vi "roboRIO v1.0 Open Relay.vi"(7 "Allow multiple opens?":bool, 8 "error in (no error)":errorcluster, 10 "Channel Names":string[](array[string]), 11 "Resource name":T3 caption="RIO Device") -> (0 "error out":errorcluster, 2 "Relay Channel List":T4, 3 "myRIO Ref Out":T1)   [LabVIEW 2021]
uses:
  <vilib>/myRIO/Common/Instrument Driver Framework/roboRIO v1.0/Relay/typedefs/Relay Channels List.ctl
  <vilib>/myRIO/Common/Instrument Driver Framework/roboRIO v1.0/Relay/typedefs/Relay Channels Enum.ctl
  <vilib>/userDefined/High Color/nirio_resource_hc.ctl
  <vilib>/myRIO/Common/Instrument Driver Framework/Utilities/typedefs/myRIO v1.0 Reference.ctl
  <vilib>/myRIO/Common/Instrument Driver Framework/Utilities/typedefs/Generic FPGA Reference.ctl
  <vilib>/myRIO/Common/Instrument Driver Framework/roboRIO v1.0/Resource Manager/vis/roboRIO v1.0 Reserve Channel List.vi
  <vilib>/myRIO/Common/Instrument Driver Framework/roboRIO v1.0/Relay/vis/roboRIO v1.0 Build MUX Configuration Relay.vi
  <vilib>/myRIO/Common/Instrument Driver Framework/roboRIO v1.0/Resource Manager/vis/roboRIO v1.0 Reserve Channel.vi
  <vilib>/myRIO/Common/Instrument Driver Framework/roboRIO v1.0/Resource Manager/vis/roboRIO v1.0 Unreserve Channel.vi
  <vilib>/myRIO/Common/Instrument Driver Framework/roboRIO v1.0/Resource Manager/vis/roboRIO v1.0 Build Mutex Name.vi
  <vilib>/Utility/VariantDataType/GetNumericInfo.vi
  <vilib>/Utility/error.llb/Error Cluster From Error Code.vi
  <vilib>/myRIO/Common/Instrument Driver Framework/Utilities/vis/IO Manager.vi
  <vilib>/myRIO/Common/Instrument Driver Framework/Utilities/vis/Configuration Manager.vi
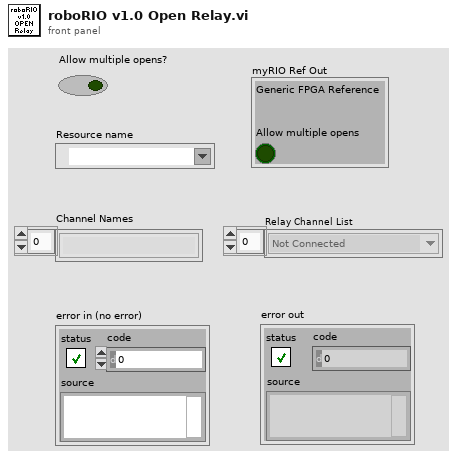
[diagram p1: front panel]
types:
  T1 = typedef "myRIO v1.0 Reference.ctl" = cluster{"Generic FPGA Reference":T2, "Allow multiple opens":bool}
  T2 = typedef "Generic FPGA Reference.ctl" = refnum<k20>
  T3 = typedef "nirio_resource_hc.ctl" = tag
  T4 = typedef "Relay Channels List.ctl" = T5[]
  T5 = typedef "Relay Channels Enum.ctl" = enum16{"Not Connected", "RELAY/RELAY0", "RELAY/RELAY1", "RELAY/RELAY2", "RELAY/RELAY3"}
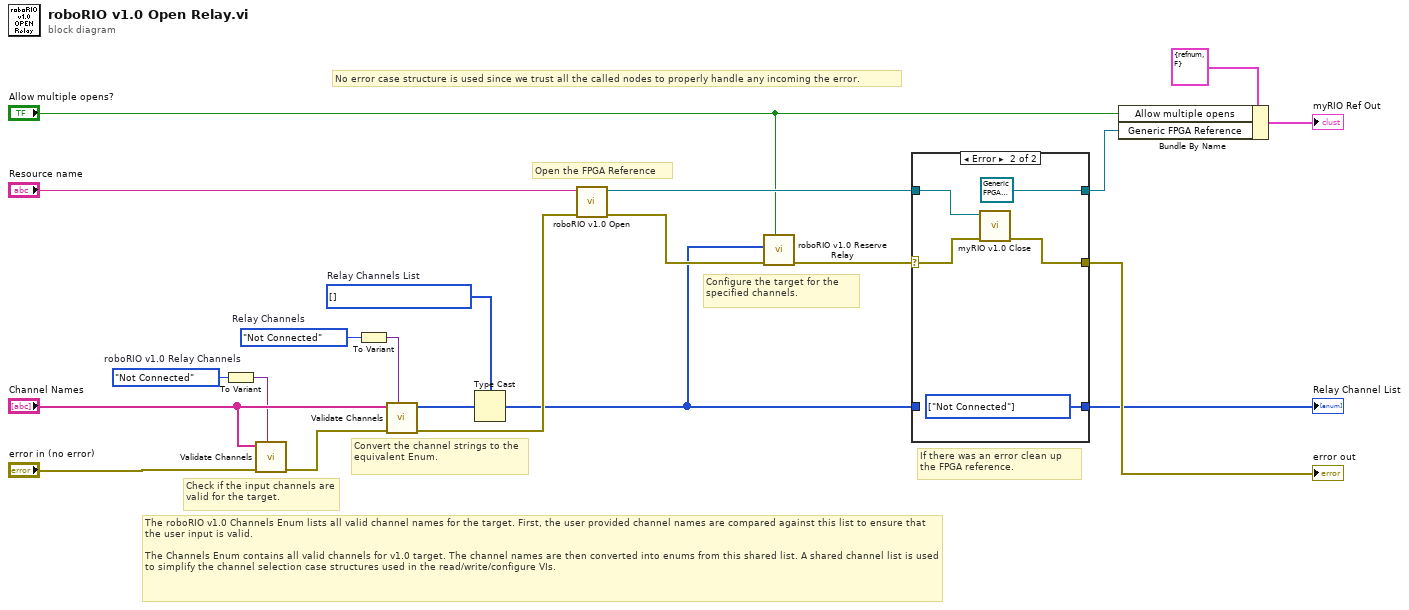
[diagram p0: block diagram]
diagram:
  w2 = Relay_Channels_Enum."Not Connected"  # Relay Channels
  w1 = Relay_Channels_Enum."Not Connected"  # roboRIO v1.0 Relay Channels
  w15 = T4 [] items=["Not Connected", "RELAY/RELAY0", "RELAY/RELAY1", "RELAY/RELAY2", "RELAY/RELAY3"]  # Relay Channels List
  # "The roboRIO v1.0 Channels Enum lists all valid channel names for the target. First, the user provided channel names are compared against this list to ensure that the user input is valid.\n\nThe Channels Enum contains all valid channels for v1.0 target. The channel names are then converted into enums from this shared list. A shared channel list is used to simplify the channel selection case structures used in the read/write/configure VIs."
  # "If there was an error clean up the FPGA reference."
  # "Configure the target for the specified channels."
  # "Open the FPGA Reference"
  # "No error case structure is used since we trust all the called nodes to properly handle any incoming the error."
  # "Convert the channel strings to the equivalent Enum."
  # "Check if the input channels are valid for the target."
  n1 = To Variant(anything=w1) -> (Variant=w3:variant)
  n2 = call <vilib>:"Validate Channels.vi"("Channels Enum Variant"=w3, "error in (no error)"="error in (no error)", "Channel Names"="Channel Names") -> ("error out"=w20:errorcluster)  [unwired: 7 in, 1 out]
  n3 = To Variant(anything=w2) -> (Variant=w4:variant)
  n4 = call <vilib>:"Validate Channels.vi"("Channels Enum Variant"=w4, "error in (no error)"=w20, "Channel Names"="Channel Names") -> ("error out"=w16:errorcluster, "Index Array"=w14:u16[])  [unwired: 7 in]
  n5 = Type Cast(type=w15, x=w14) -> (*(type *) &x=w10:T4)
  n6 = call <vilib>:"roboRIO v1.0 Open.vi"("error in (no error)"=w16, "Resource name"="Resource name") -> ("error out"=w13:errorcluster, "myRIO FPGA Ref Out"=w11:T2)  [unwired: 8 in]
  n7 = call <vilib>:"roboRIO v1.0 Reserve Relay.vi"("Allow multiple opens?"="Allow multiple opens?", "error in (no error)"=w13, "Relay Channel List"=w10) -> ("error out"=w12:errorcluster)  [unwired: 8 in]
  n8 = case shown="Error" w12 {
    selector: w12 -> [w23 w29]
    tunnel: w11 -> [w24 w27]
    tunnel: [w24 T2 refnum ("roboRIO FPGA Ref Out")] -> w6
    tunnel: [w23 w28] -> w18
    tunnel: w10 -> [w22 _]
    tunnel: [w22 w25] -> w9
    frame No Error {
    }
    frame Error {
      w25 = T4 [enum."Not Connected"] items=["Not Connected", "RELAY/RELAY0", "RELAY/RELAY1", "RELAY/RELAY2", "RELAY/RELAY3"] ("DIO Channels List")
      n9 = call <vilib>:"myRIO v1.0 Close.vi"("error in (no error)"=w29, "myRIO FPGA Ref In"=w27) -> ("error out"=w28:errorcluster)  [unwired: 9 in]
    }
  }
  "Relay Channel List" <- w9
  "error out" <- w18
  n10 = Bundle By Name(cluster=T1 {"Generic FPGA Reference"=refnum, "Allow multiple opens"=FALSE} ("myRIO Hardware Reference"), "Allow multiple opens"="Allow multiple opens?", "Generic FPGA Reference"=w6) -> (→"myRIO Ref Out":T1)
